vi "ProbeStationId.vi"() -> ()   [LabVIEW 2012]
panel:
  in  "ProbeStationId":i32
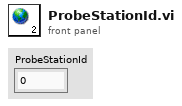
[diagram p1: front panel]
diagram:
